vi "LamdaShiftFlow.vi"() -> ()   [LabVIEW 2022 SP3]
panel:
  out "prf":dbl
  out "half lamda time":dbl
  in  "final time ms":dbl=25.0
  out "Waveform Graph":cluster{"x/y":dbl, dbl, dbl[][]}(graph)
  in  "steps":i32=100
  in  "velocity mm/ms":dbl=0.06400000000000006
  out "lamda (um)":dbl
  in  "fc MHz":dbl=15.0
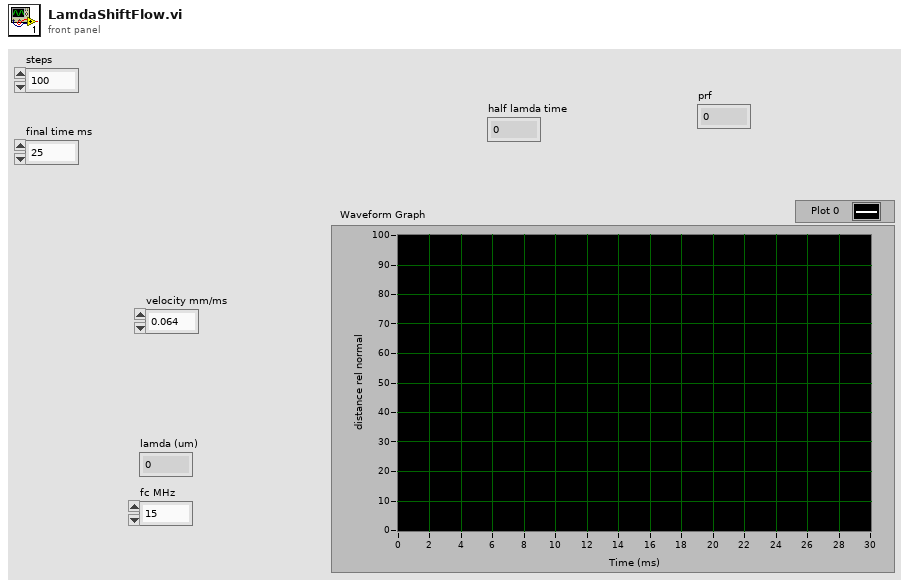
[diagram p1: front panel]
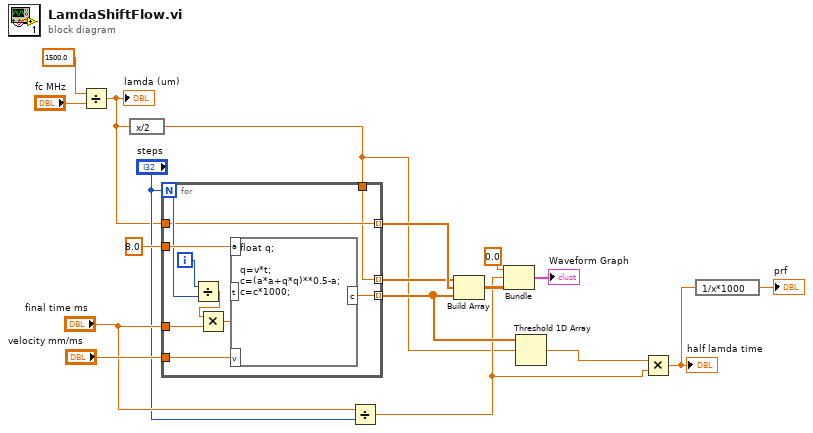
[diagram p0: block diagram]
diagram:
  n1 = Divide(x=1500.0, y="fc MHz") -> (x/y=w7:dbl)
  "lamda (um)" <- w7
  n2 = expression code="x/2"(w7) -> (w4:dbl)
  n3 = for {
    N: "steps" -> [w26]
    tunnel: 8.0 ("input variable") -> [w28]
    tunnel: "velocity mm/ms" -> [w27]
    tunnel: [w24] -> w6 mode=indexing
    tunnel: [w23] -> w14 mode=indexing
    tunnel: w7 -> [w23]
    tunnel: "final time ms" -> [w20]
    tunnel: [w19] -> w13 mode=indexing
    tunnel: w4 -> [w19]
    i -> [w25]
    n4 = Divide(x=w25, y=w26) -> (x/y=w22:dbl)
    n5 = Multiply(x=w22, y=w20) -> (x*y=w21:dbl)
    n6 = formula code="float q;\n\nq=v*t;\nc=(a*a+q*q)**0.5-a;\nc=c*1000;"("a"=w28, "v"=w27, "t"=w21) -> ("c"=w24:dbl)
  }
  n7 = Divide(x="final time ms", y="steps") -> (x/y=w5:dbl)
  n8 = Build Array(w13, w14, w6) -> (w12:dbl[][])
  n9 = Bundle("x/y"=0.0, w5, w12) -> (→"Waveform Graph":cluster{"x/y":dbl, dbl, dbl[][]})  [unwired: 1 in]
  n10 = Threshold 1D Array(2:w4, 3:w6) -> (0:w3:dbl)  [unwired: 1 in]
  n11 = Multiply(x=w3, y=w5) -> (x*y=w2:dbl)
  "half lamda time" <- w2
  n12 = expression code="1/x*1000"(w2) -> (→"prf":dbl)
